vi "figureTurn.vi"(8 "Total Y":dbl, 9 "Total X":dbl, 10 "Center Y":dbl, 11 "Center X":dbl) -> ()   [LabVIEW 2019]
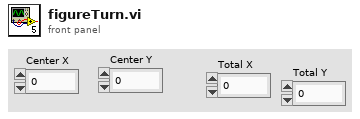
[diagram p1: front panel]
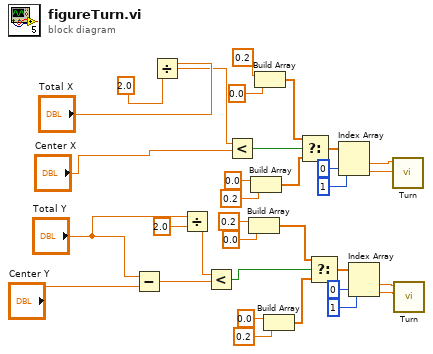
[diagram p0: block diagram]
diagram:
  n1 = Subtract(x="Total Y", y="Center Y") -> (x-y=w30:dbl)
  n2 = Divide(x="Total X", y=2.0) -> (x/y=w23:dbl)
  n3 = Divide(x="Total Y", y=2.0) -> (x/y=w27:dbl)
  n4 = Less?(x=w27, y=w30) -> (x < y?=w26:bool)
  n5 = Less?(x=w23, y="Center X") -> (x < y?=w25:bool)
  n6 = Build Array(0.2 ("element"), 0.0 ("element")) -> (w14:dbl[])
  n7 = Build Array(0.0 ("element"), 0.2 ("element")) -> (w21:dbl[])
  n8 = Build Array(0.2 ("element"), 0.0 ("element")) -> (w22:dbl[])
  n9 = Build Array(0.0 ("element"), 0.2 ("element")) -> (w11:dbl[])
  n10 = Select(t=w22, s=w25, f=w21) -> (s? t:f=w10:dbl[])
  n11 = Select(t=w14, s=w26, f=w11) -> (s? t:f=w9:dbl[])
  n12 = Index Array(array=w10, index #1=0 ("index"), index #2=1 ("index")) -> (element #1=w8:dbl, element #2=w7:dbl)
  n13 = Index Array(array=w9, index #1=0 ("index"), index #2=1 ("index")) -> (element #1=w6:dbl, element #2=w5:dbl)
  n14 = call "Turn.vi"("Right Setpoint"=w7, "Left Setpoint"=w8) -> ()  [unwired: 10 in]
  n15 = call "Turn.vi"("Right Setpoint"=w5, "Left Setpoint"=w6) -> ()  [unwired: 10 in]
